vi "Create All Message Queues.vi"(8 "error in":errorcluster) -> (0 "error out":errorcluster, 3 "Queues":T1)   [LabVIEW 2015, in "Message Queue.lvlib"]
doc: "Creates and initializes message queues"
uses:
  Message Queue.lvlib
  All Message Queues.ctl
  Message Cluster.ctl
  Enqueue Message (Single).vi
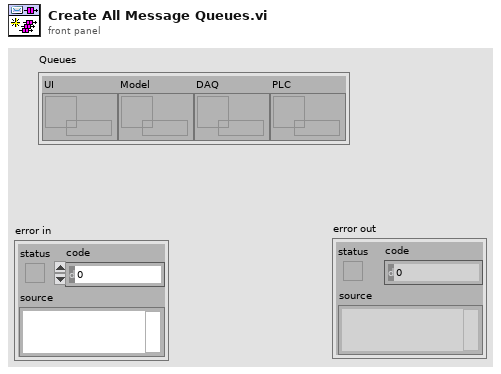
[diagram p1: front panel]
types:
  T1 = typedef "Message Queue.lvlib/All Message Queues.ctl" = cluster{"UI":refnum<queue>, "Model":refnum<queue>, "DAQ":refnum<queue>, "PLC":refnum<queue>}
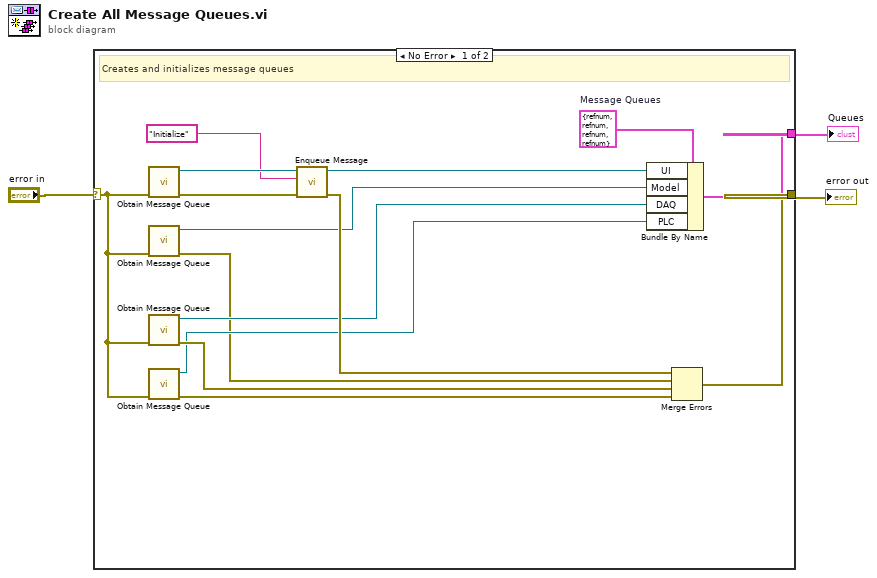
[diagram p0: block diagram]
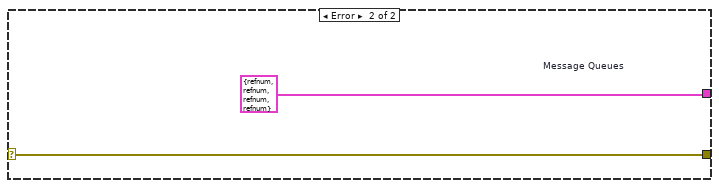
[diagram p2: hidden frame]
diagram:
  n1 = case shown="No Error" "error in" {
    selector: "error in" -> [w11 w20]
    tunnel: [w12 w20] -> w3
    tunnel: [w17 w19] -> w2
    frame No Error {
      w18 = T1 {"UI"=refnum, "Model"=refnum, "DAQ"=refnum, "PLC"=refnum}  # Message Queues
      # "Creates and initializes message queues"
      n2 = call "Obtain Message Queue.vi"("error in (no error)"=w11) -> ("error out"=w16:errorcluster, "Message Queue"=w15:refnum<queue>)  [unwired: 9 in]
      n3 = call "Obtain Message Queue.vi"("error in (no error)"=w11) -> ("error out"=w5:errorcluster, "Message Queue"=w4:refnum<queue>)  [unwired: 9 in]
      n4 = call "Obtain Message Queue.vi"("error in (no error)"=w11) -> ("error out"=w8:errorcluster, "Message Queue"=w9:refnum<queue>)  [unwired: 9 in]
      n5 = call "Obtain Message Queue.vi"("error in (no error)"=w11) -> ("error out"=w6:errorcluster, "Message Queue"=w7:refnum<queue>)  [unwired: 9 in]
      n6 = call-poly "Enqueue Message.vi"("error in (no error)"=w16, "Message"="Initialize", "Message Queue"=w15) -> ("error out"=w13:errorcluster, "dup Message Queue"=w14:refnum<queue>)  [unwired: 7 in]
      n7 = Bundle By Name(cluster=w18, "UI"=w14, "Model"=w4, "DAQ"=w9, "PLC"=w7) -> (w17:T1)
      n8 = Merge Errors(w13, w5, w8, w6) -> (w12:errorcluster)
    }
    frame Error {
      w19 = T1 {"UI"=refnum, "Model"=refnum, "DAQ"=refnum, "PLC"=refnum}  # Message Queues
    }
  }
  "Queues" <- w2
  "error out" <- w3
